vi "日志信息出发送队列 (子VI).vi"(11 "queue out":refnum<queue>) -> (0 "错误输出":errorcluster)   [LabVIEW 2016, in "数据传输系统-03.lvlib"]
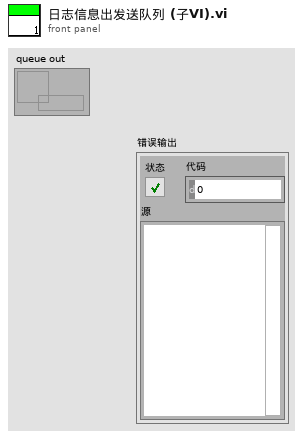
[diagram p1: front panel]
types:
  T1 = enum16{"空白测试", "跨度核查", "标样核查", "加标回收", "平行样", "集成干预"}
  T2 = typedef "数据传输系统-03.lvlib/应用环境.ctl" = enum16{"STD", "GB212", "婉仪平台"}
  T3 = cluster{"氨氮零点核查索引起始时间":string, "总磷零点核查索引起始时间":string, "总氮零点核查索引起始时间":string, "CODMn零点核查索引起始时间":string, "CODCr零点核查索引起始时间":string, "亚硝酸盐零点核查索引起始时间":string, "硫化物零点核查索引起始时间":string, "ORP零点核查索引起始时间":string, "氟化物零点核查索引起始时间":string, "挥发酚零点核查索引起始时间":string}
  T4 = cluster{"数组[0]":string, "数组[1]":string, "数组[2]":string, "数组[3]":string, "数组[4]":string, "数组[5]":string, "数组[6]":string, "数组[7]":string, "数组[8]":string, "数组[9]":string}
  T5 = cluster{"PH":string[][], "CODCr":string[][], "氨氮":string[][], "CODMn":string[][], "总氮":string[][], "总磷":string[][], "电导率":string[][], "水温":string[][], "COD":string[][], "DO":string[][], "浊度":string[][], "叶绿素":string[][], "藻密度":string[][], "铜":string[][], "盐度":string[][], "水位":string[][], "流速":string[][], "方向":string[][], "瞬时流量":string[][], "累积流量":string[][], "正累积流量":string[][], "负累积流量":string[][], "亚硝酸盐":string[][], "硫化物":string[][], "ORP":string[][], "铅":string[][], "镉":string[][], "锌":string[][], "镍":string[][], "锰":string[][], "汞":string[][], "气温":string[][], "气压":string[][], "风速":string[][], "风向":string[][], "空气温度":string[][], "相对湿度":string[][], "分钟雨量":string[][], "小时雨量":string[][], "日雨量":string[][], "累积雨量":string[][], "盐度":string[][], "磷酸盐":string[][], "硝氮":string[][], "氟化物":string[][], "挥发酚":string[][], "氯化物":string[][], "蓝绿藻":string[][], "余氯":string[][], "综合生物毒性":string[][], "水深":string[][]}
  T6 = cluster{"氨氮跨度核查索引起始时间":string, "总磷跨度核查索引起始时间":string, "总氮跨度核查索引起始时间":string, "CODMn跨度核查索引起始时间":string, "CODCr跨度核查索引起始时间":string, "亚硝酸盐跨度核查索引起始时间":string, "硫化物跨度核查索引起始时间":string, "ORP跨度核查索引起始时间":string, "氟化物跨度核查索引起始时间":string, "挥发酚跨度核查索引起始时间":string}
  T7 = cluster{"氨氮标样核查索引起始时间":string, "总磷标样核查索引起始时间":string, "总氮标样核查索引起始时间":string, "CODMn标样核查索引起始时间":string, "CODCr标样核查索引起始时间":string, "DO标样核查索引起始时间":string, "PH标样核查索引起始时间":string, "比电导率标样核查索引起始时间":string, "水温标样核查索引起始时间":string, "浊度标样核查索引起始时间":string, "叶绿素a标样核查索引起始时间":string, "藻密度标样核查索引起始时间":string, "亚硝酸盐标样核查索引起始时间":string, "硫化物标样核查索引起始时间":string, "ORP标样核查索引起始时间":string, "氟化物标样核查索引起始时间":string, "挥发酚标样核查索引起始时间":string, "氯化物标样核查索引起始时间":string}
  T8 = cluster{"数组[0]":string, "数组[1]":string, "数组[2]":string, "数组[3]":string, "数组[4]":string, "数组[5]":string, "数组[6]":string, "数组[7]":string, "数组[8]":string, "数组[9]":string, "数组[10]":string, "数组[11]":string, "数组[12]":string, "数组[13]":string, "数组[14]":string, "数组[15]":string, "数组[16]":string, "数组[17]":string}
  T9 = cluster{"氨氮加标回收索引起始时间":string, "总磷加标回收索引起始时间":string, "总氮加标回收索引起始时间":string, "CODMn加标回收索引起始时间":string, "CODCr加标回收索引起始时间":string, "氟化物加标回收索引起始时间":string, "挥发酚加标回收索引起始时间":string}
  T10 = cluster{"[0]":string, "[1]":string, "[2]":string, "[3]":string, "[4]":string, "[5]":string, "[6]":string}
  T11 = cluster{"氨氮平行样索引起始时间":string, "总磷平行样索引起始时间":string, "总氮平行样索引起始时间":string, "CODMn平行样索引起始时间":string, "CODCr平行样索引起始时间":string, "氟化物平行样索引起始时间":string, "挥发酚平行样索引起始时间":string}
  T12 = cluster{"氨氮集成干预索引起始时间":string, "总磷集成干预索引起始时间":string, "总氮集成干预索引起始时间":string, "CODMn集成干预索引起始时间":string, "CODCr集成干预索引起始时间":string, "DO集成干预索引起始时间":string, "PH集成干预索引起始时间":string, "比电导率集成干预索引起始时间":string, "水温集成干预索引起始时间":string, "浊度集成干预索引起始时间":string, "叶绿素a集成干预索引起始时间":string, "藻密度集成干预索引起始时间":string, "亚硝酸盐集成干预索引起始时间":string, "硫化物集成干预索引起始时间":string, "ORP集成干预索引起始时间":string, "氟化物集成干预索引起始时间":string, "挥发酚集成干预索引起始时间":string, "氯化物集成干预索引起始时间":string}
  T13 = cluster{"[0]":string, "[1]":string, "[2]":string, "[3]":string, "[4]":string, "[5]":string, "[6]":string, "[7]":string, "[8]":string, "[9]":string, "[10]":string, "[11]":string, "[12]":string, "[13]":string, "[14]":string, "[15]":string, "[16]":string, "[17]":string}
  T14 = cluster{"氨氮仪器日志索引起始时间":string, "总磷仪器日志索引起始时间":string, "总氮仪器日志索引起始时间":string, "CODMn仪器日志索引起始时间":string, "CODCr仪器日志索引起始时间":string, "系统仪器日志索引起始时间":string, "氟化物仪器日志索引起始时间":string, "挥发酚仪器日志索引起始时间":string}
  T15 = cluster{"[0]":string, "[1]":string, "[2]":string, "[3]":string, "[4]":string, "[5]":string, "[6]":string, "[7]":string}
  T16 = cluster{"氨氮报警信息索引起始时间":string, "总磷报警信息索引起始时间":string, "总氮报警信息索引起始时间":string, "CODMn报警信息索引起始时间":string, "CODCr报警信息索引起始时间":string, "DO报警信息索引起始时间":string, "PH报警信息索引起始时间":string, "比电导率报警信息索引起始时间":string, "水温报警信息索引起始时间":string, "浊度报警信息索引起始时间":string, "叶绿素报警信息索引起始时间":string, "系统报警信息索引起始时间":string, "氟化物报警信息索引起始时间":string, "挥发酚报警信息索引起始时间":string}
  T17 = cluster{"[0]":string, "[1]":string, "[2]":string, "[3]":string, "[4]":string, "[5]":string, "[6]":string, "[7]":string, "[8]":string, "[9]":string, "[10]":string, "[11]":string, "[12]":string, "[13]":string}
  T18 = cluster{"氨氮仪器参数索引起始时间":string, "总磷仪器参数索引起始时间":string, "总氮仪器参数索引起始时间":string, "CODMn仪器参数索引起始时间":string, "CODCr仪器参数索引起始时间":string, "DO仪器参数索引起始时间":string, "PH仪器参数索引起始时间":string, "比电导率仪器参数索引起始时间":string, "水温仪器参数索引起始时间":string, "浊度仪器参数索引起始时间":string, "叶绿素a仪器参数索引起始时间":string, "藻密度仪器参数索引起始时间":string, "ORP仪器参数索引起始时间":string, "氟化物仪器参数索引起始时间":string, "挥发酚仪器参数索引起始时间":string}
  T19 = cluster{"[0]":string, "[1]":string, "[2]":string, "[3]":string, "[4]":string, "[5]":string, "[6]":string, "[7]":string, "[8]":string, "[9]":string, "[10]":string, "[11]":string, "[12]":string, "[13]":string, "[14]":string}
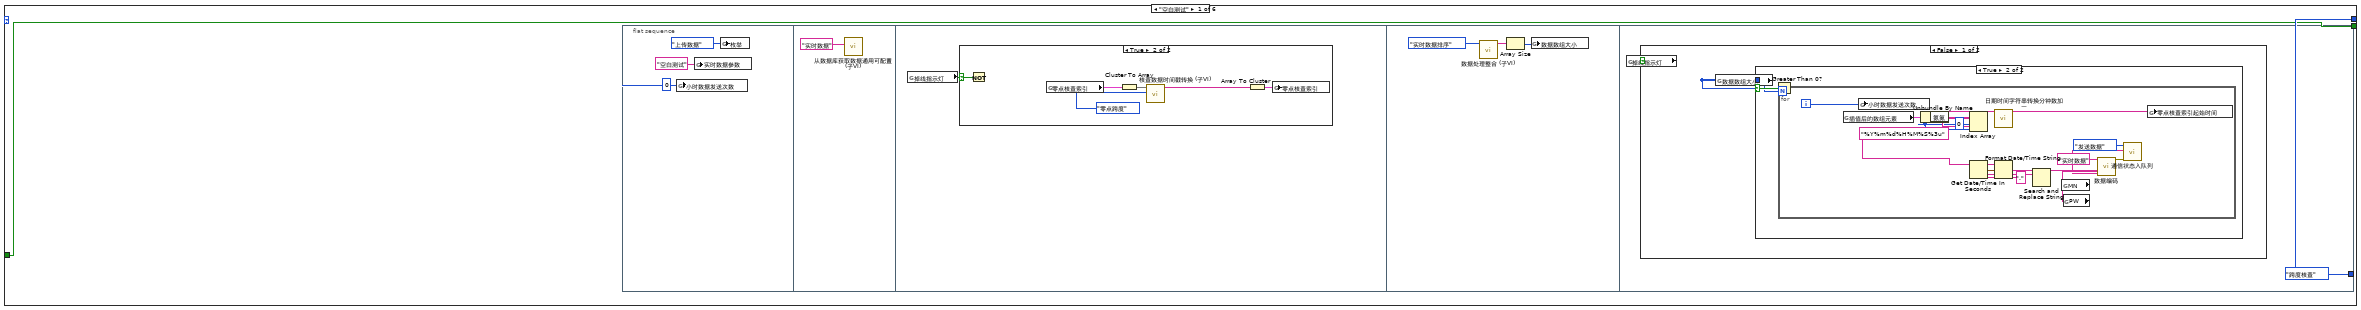
[diagram p2: hidden frame]
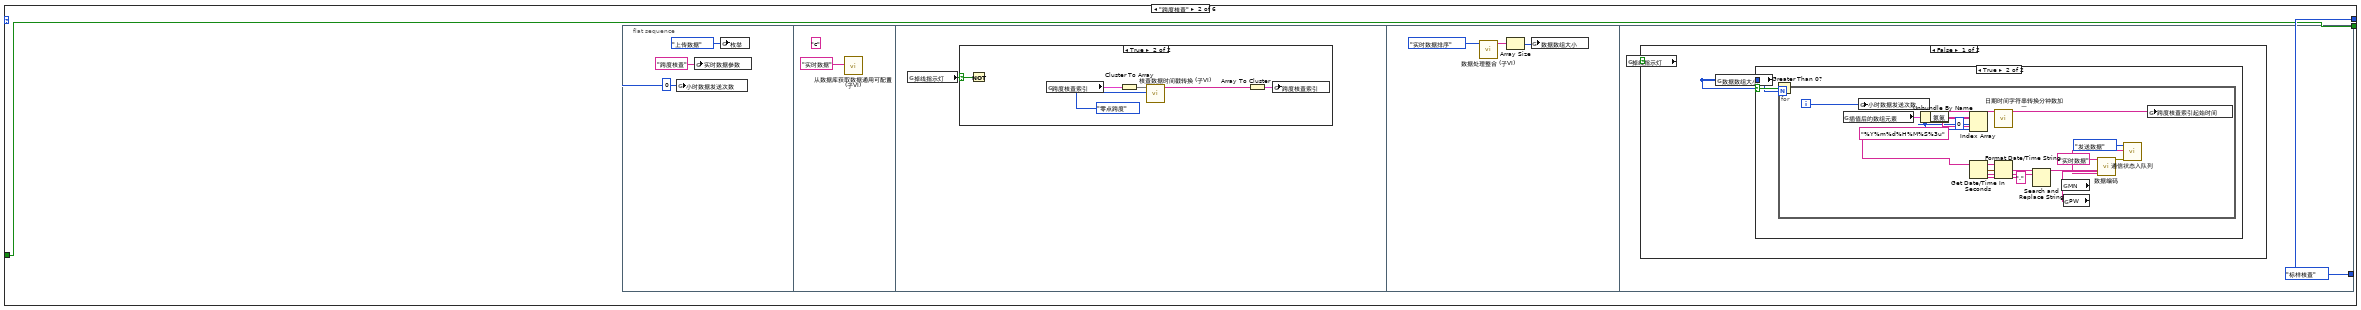
[diagram p6: hidden frame]
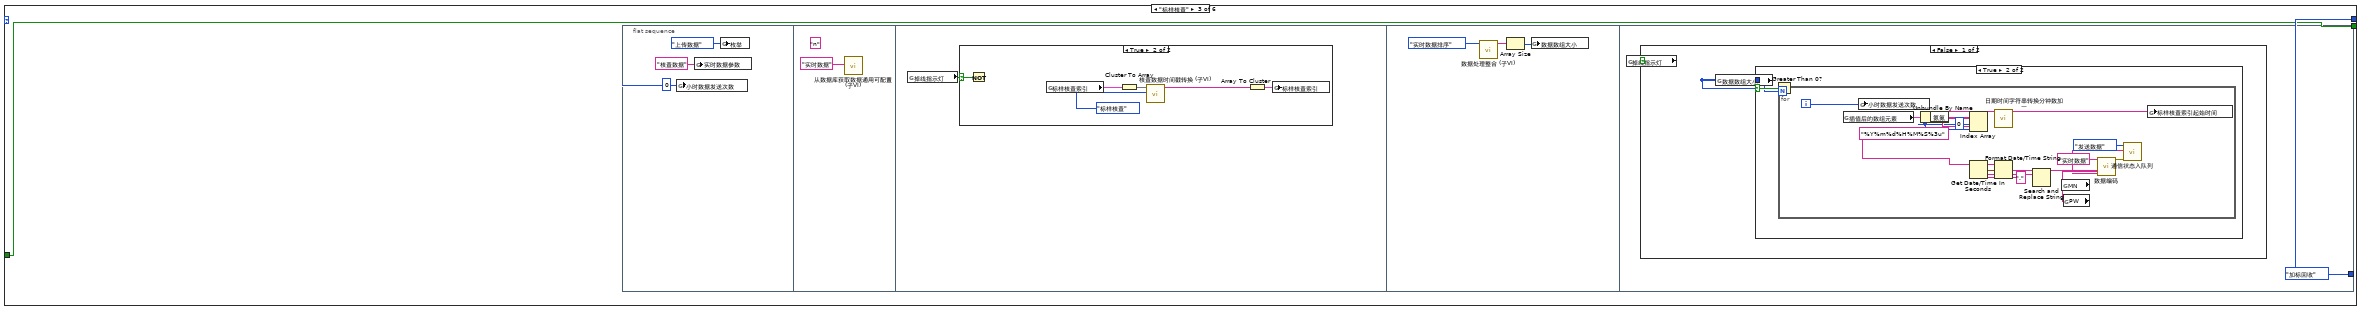
[diagram p10: hidden frame]
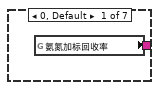
[diagram p15: hidden frame]
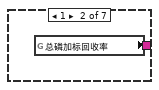
[diagram p16: hidden frame]
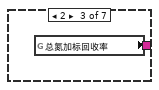
[diagram p17: hidden frame]
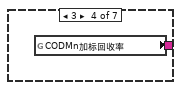
[diagram p18: hidden frame]
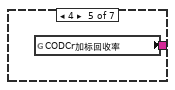
[diagram p19: hidden frame]
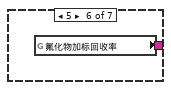
[diagram p20: hidden frame]
diagram:
  n1 = while "While循环" {
    shift-right: [w12] -> _
    shift-left: "质控数据" ("组合框") -> [w13]
    tunnel: [errorcluster {"status"=FALSE, "code"=0, "source"=""} ("错误输出")] -> w3
    tunnel: "queue out" -> [w9]
    stop <- w10 stop-if-true
    # "所有的主动上传数据都是有数据才会上传"
    n2 = Get Queue Status(queue=w9, return elements? (F)=TRUE ("返回元素？(F)")) -> (elements=w8:string[])  [unwired: 1 in, 7 out]
    n3 = Index Array(array=w8) -> (element=w7:string)  [unwired: 1 in]
    n4 = Equal?(x=w7, y="反控命令" ("元素")) -> (x = y?=w5:bool)
    n5 = case shown="\"质控数据\"" w13 {
      tunnel: [w23 w328 "系统状态" ("组合框") w431 "测量周期" ("组合框") "超标留样" ("组合框") "报警信息" ("组合框") w576 w643 "环境参数" ("组合框") "环境参数" ("组合框")] -> w12
      tunnel: [w14 w327 w385 w429 w455 w489 w554 w575 w642 w689 TRUE] -> w10
      tunnel: w5 -> [w14 w327 w385 w429 w455 w489 w554 w575 w642 w689 _]
      frame "质控数据" {
        n6 = global read "断电保存全局.vi" "数据组合发送"() -> (w18:bool)
        n7 = global read "断电保存全局.vi" "数据发送协议"() -> (w21:enum16{"2005-212协议", "2017-212协议"})
        n8 = Not(x=w18) -> (.not. x?=w17:bool)
        n9 = Equal?(x=w21, y=enum16{"2005-212协议", "2017-212协议"}."2017-212协议" ("数据发送协议")) -> (x = y?=w19:bool)
        n10 = And(x=w17, y=w19) -> (x .and. y?=w16:bool)
        n11 = case shown="True" w16 {
          tunnel: [T1."空白测试" T1."加标回收"] -> w15
          frame False {
          }
          frame True {
          }
        }
        n12 = while {
          shift-right: [w27] -> _
          shift-left: w15 -> [w28]
          tunnel: w14 -> [w24]
          stop <- w25 stop-if-true
          n13 = case shown="\"加标回收\"" w28 {
            tunnel: [w29 w67 w105 w143 w204 TRUE] -> w25
            tunnel: [w30 w68 w106 w144 w205 w258] -> w27
            tunnel: w24 -> [w29 w67 w105 w143 w204 _]
            frame "空白测试" {
              n14 = flat-sequence {
                tunnel: [T1."跨度核查"] -> w30
                frame #0 {
                  n15 = global write "全局 小时数据发送次数.vi" "小时数据发送次数"(0 ("小时数据发送次数")) -> ()
                  n16 = global write "全局 实时数据参数.vi" "实时数据参数"("空白测试") -> ()
                  n17 = global write "全局1.vi" "枚举"(enum16{"返回请求应答", "上传数据", "返回执行结果"}."上传数据" ("枚举")) -> ()
                }
                frame #1 {
                  n18 = call "从数据库获取数据通用可配置(子VI).vi"("table输入"="实时数据" ("新元素/子数组")) -> ()  [unwired: 9 in, 2 out]
                }
                frame #2 {
                  n19 = global read "全局 数据发送重叠.vi" "掉线指示灯"() -> (w36:bool)
                  n20 = Not(x=w36) -> (.not. x?=w35:bool)
                  n21 = case shown="True" w35 {
                    frame False {
                    }
                    frame True {
                      n22 = global read "全局 时间2.vi" "零点核查索引"() -> (w41:T3)
                      n23 = Cluster To Array(cluster=w41) -> (array=w39:string[])
                      n24 = call "核查数据时间戳转换 (子VI).vi"("枚举"=enum16{"零点跨度", "标样核查"}."零点跨度", "核查索引"=w39) -> ("数组"=w38:string[])  [unwired: 9 in]
                      n25 = Array To Cluster(array=w38) -> (cluster=w40:T4)
                      n26 = global write "全局 时间2.vi" "零点核查索引"(w40) -> ()
                    }
                  }
                }
                frame #3 {
                  n27 = call "数据处理整合 (子VI).vi"("枚举"=enum16{"实时数据排序", "小时数据排序"}."实时数据排序") -> ("已排序的数组"=w44:string[])  [unwired: 10 in]
                  n28 = Array Size(array=w44) -> (size(s)=w43:i32)
                  n29 = global write "全局 数据数组大小.vi" "数据数组大小"(w43) -> ()
                }
                frame #4 {
                  n30 = global read "全局 数据发送重叠.vi" "掉线指示灯"() -> (w46:bool)
                  n31 = case shown="False" w46 {
                    frame False {
                      n32 = global read "全局 数据数组大小.vi" "数据数组大小"() -> (w47:i32)
                      n33 = Greater Than 0?(x=w47) -> (x > 0?=w48:bool)
                      n34 = case shown="True" w48 {
                        tunnel: w47 -> [_ w49]
                        frame False {
                        }
                        frame True {
                          n35 = for {
                            N: w49 -> [_]
                            i -> [w52]
                            w61 = 0 ("禁用的索引 (列)")
                            n36 = global read "插值后的新数组.vi" "插值后的数组元素"() -> (w65:T5)
                            n37 = global write "全局 小时数据发送次数.vi" "小时数据发送次数"(w52) -> ()
                            n38 = Unbundle By Name(w65) -> ("氨氮"=w64:string[][])
                            n39 = Index Array(array=w64, index (row)=w61, index (col)=w61) -> (element=w63:string)
                            n40 = Get Date/Time In Seconds() -> (seconds since 1Jan1904=w56:timestamp)
                            n41 = call "日期时间字符串转换分钟数加一.vi"("data[0]"=w63) -> ("日期/时间字符串"=w62:string)  [unwired: 10 in]
                            n42 = Format Date/Time String(time format string (%c)="%Y%m%d%H%M%S%3u" ("时间格式字符串(%c)"), seconds (now)=w56) -> (date/time string=w55:string)  [unwired: 1 in]
                            n43 = Search and Replace String(input string=w55, search string="." ("搜索字符串")) -> (result string=w53:string)  [unwired: 6 in, 3 out]
                            n44 = global read "断电保存全局.vi" "MN"() -> (w60:string)
                            n45 = global read "断电保存全局.vi" "PW"() -> (w59:string)
                            n46 = call "数据编码.vi"("table输入"="实时数据" ("新元素/子数组"), "QN"=w53, "MN"=w60, "PW"=w59) -> ("错误常量"=w58:errorcluster, "通讯包字符串"=w50:string)  [unwired: 10 in]
                            n47 = call "通信状态入队列.vi"("错误输入（无错误）"=w58, "发送报文"=w50, "枚举"=enum16{"打开连接", "发送数据", "读取数据", "数据处理", "关闭连接"}."发送数据") -> ()  [unwired: 8 in, 1 out]
                            n48 = global write "全局 时间2.vi" "零点核查索引起始时间"(w62) -> ()
                          }
                        }
                      }
                    }
                    frame True {
                    }
                  }
                }
              }
            }
            frame "跨度核查" {
              n49 = flat-sequence {
                tunnel: [T1."标样核查"] -> w68
                frame #0 {
                  n50 = global write "全局 小时数据发送次数.vi" "小时数据发送次数"(0 ("小时数据发送次数")) -> ()
                  n51 = global write "全局 实时数据参数.vi" "实时数据参数"("跨度核查") -> ()
                  n52 = global write "全局1.vi" "枚举"(enum16{"返回请求应答", "上传数据", "返回执行结果"}."上传数据" ("枚举")) -> ()
                }
                frame #1 {
                  (unwired) "c" ("列队名（唯一）")
                  n53 = call "从数据库获取数据通用可配置(子VI).vi"("table输入"="实时数据" ("新元素/子数组")) -> ()  [unwired: 9 in, 2 out]
                }
                frame #2 {
                  n54 = global read "全局 数据发送重叠.vi" "掉线指示灯"() -> (w74:bool)
                  n55 = Not(x=w74) -> (.not. x?=w73:bool)
                  n56 = case shown="True" w73 {
                    frame False {
                    }
                    frame True {
                      n57 = global read "全局 时间2.vi" "跨度核查索引"() -> (w79:T6)
                      n58 = Cluster To Array(cluster=w79) -> (array=w77:string[])
                      n59 = call "核查数据时间戳转换 (子VI).vi"("枚举"=enum16{"零点跨度", "标样核查"}."零点跨度", "核查索引"=w77) -> ("数组"=w76:string[])  [unwired: 9 in]
                      n60 = Array To Cluster(array=w76) -> (cluster=w78:T4)
                      n61 = global write "全局 时间2.vi" "跨度核查索引"(w78) -> ()
                    }
                  }
                }
                frame #3 {
                  n62 = call "数据处理整合 (子VI).vi"("枚举"=enum16{"实时数据排序", "小时数据排序"}."实时数据排序") -> ("已排序的数组"=w82:string[])  [unwired: 10 in]
                  n63 = Array Size(array=w82) -> (size(s)=w81:i32)
                  n64 = global write "全局 数据数组大小.vi" "数据数组大小"(w81) -> ()
                }
                frame #4 {
                  n65 = global read "全局 数据发送重叠.vi" "掉线指示灯"() -> (w84:bool)
                  n66 = case shown="False" w84 {
                    frame False {
                      n67 = global read "全局 数据数组大小.vi" "数据数组大小"() -> (w85:i32)
                      n68 = Greater Than 0?(x=w85) -> (x > 0?=w86:bool)
                      n69 = case shown="True" w86 {
                        tunnel: w85 -> [_ w87]
                        frame False {
                        }
                        frame True {
                          n70 = for {
                            N: w87 -> [_]
                            i -> [w90]
                            w99 = 0 ("禁用的索引 (列)")
                            n71 = global read "插值后的新数组.vi" "插值后的数组元素"() -> (w103:T5)
                            n72 = global write "全局 小时数据发送次数.vi" "小时数据发送次数"(w90) -> ()
                            n73 = Unbundle By Name(w103) -> ("氨氮"=w102:string[][])
                            n74 = Index Array(array=w102, index (row)=w99, index (col)=w99) -> (element=w101:string)
                            n75 = Get Date/Time In Seconds() -> (seconds since 1Jan1904=w94:timestamp)
                            n76 = call "日期时间字符串转换分钟数加一.vi"("data[0]"=w101) -> ("日期/时间字符串"=w100:string)  [unwired: 10 in]
                            n77 = Format Date/Time String(time format string (%c)="%Y%m%d%H%M%S%3u" ("时间格式字符串(%c)"), seconds (now)=w94) -> (date/time string=w93:string)  [unwired: 1 in]
                            n78 = Search and Replace String(input string=w93, search string="." ("搜索字符串")) -> (result string=w91:string)  [unwired: 6 in, 3 out]
                            n79 = global read "断电保存全局.vi" "MN"() -> (w98:string)
                            n80 = global read "断电保存全局.vi" "PW"() -> (w97:string)
                            n81 = call "数据编码.vi"("table输入"="实时数据" ("新元素/子数组"), "QN"=w91, "MN"=w98, "PW"=w97) -> ("错误常量"=w96:errorcluster, "通讯包字符串"=w88:string)  [unwired: 10 in]
                            n82 = call "通信状态入队列.vi"("错误输入（无错误）"=w96, "发送报文"=w88, "枚举"=enum16{"打开连接", "发送数据", "读取数据", "数据处理", "关闭连接"}."发送数据") -> ()  [unwired: 8 in, 1 out]
                            n83 = global write "全局 时间2.vi" "跨度核查索引起始时间"(w100) -> ()
                          }
                        }
                      }
                    }
                    frame True {
                    }
                  }
                }
              }
            }
            frame "标样核查" {
              n84 = flat-sequence {
                tunnel: [T1."加标回收"] -> w106
                frame #0 {
                  n85 = global write "全局 小时数据发送次数.vi" "小时数据发送次数"(0 ("小时数据发送次数")) -> ()
                  n86 = global write "全局 实时数据参数.vi" "实时数据参数"("核查数据") -> ()
                  n87 = global write "全局1.vi" "枚举"(enum16{"返回请求应答", "上传数据", "返回执行结果"}."上传数据" ("枚举")) -> ()
                }
                frame #1 {
                  (unwired) "n" ("列队名（唯一）")
                  n88 = call "从数据库获取数据通用可配置(子VI).vi"("table输入"="实时数据" ("新元素/子数组")) -> ()  [unwired: 9 in, 2 out]
                }
                frame #2 {
                  n89 = global read "全局 数据发送重叠.vi" "掉线指示灯"() -> (w112:bool)
                  n90 = Not(x=w112) -> (.not. x?=w111:bool)
                  n91 = case shown="True" w111 {
                    frame False {
                    }
                    frame True {
                      n92 = global read "全局 时间2.vi" "标样核查索引"() -> (w117:T7)
                      n93 = Cluster To Array(cluster=w117) -> (array=w115:string[])
                      n94 = call "核查数据时间戳转换 (子VI).vi"("枚举"=enum16{"零点跨度", "标样核查"}."标样核查", "核查索引"=w115) -> ("数组"=w114:string[])  [unwired: 9 in]
                      n95 = Array To Cluster(array=w114) -> (cluster=w116:T8)
                      n96 = global write "全局 时间2.vi" "标样核查索引"(w116) -> ()
                    }
                  }
                }
                frame #3 {
                  n97 = call "数据处理整合 (子VI).vi"("枚举"=enum16{"实时数据排序", "小时数据排序"}."实时数据排序") -> ("已排序的数组"=w120:string[])  [unwired: 10 in]
                  n98 = Array Size(array=w120) -> (size(s)=w119:i32)
                  n99 = global write "全局 数据数组大小.vi" "数据数组大小"(w119) -> ()
                }
                frame #4 {
                  n100 = global read "全局 数据发送重叠.vi" "掉线指示灯"() -> (w122:bool)
                  n101 = case shown="False" w122 {
                    frame False {
                      n102 = global read "全局 数据数组大小.vi" "数据数组大小"() -> (w123:i32)
                      n103 = Greater Than 0?(x=w123) -> (x > 0?=w124:bool)
                      n104 = case shown="True" w124 {
                        tunnel: w123 -> [_ w125]
                        frame False {
                        }
                        frame True {
                          n105 = for {
                            N: w125 -> [_]
                            i -> [w128]
                            w137 = 0 ("禁用的索引 (列)")
                            n106 = global read "插值后的新数组.vi" "插值后的数组元素"() -> (w141:T5)
                            n107 = global write "全局 小时数据发送次数.vi" "小时数据发送次数"(w128) -> ()
                            n108 = Unbundle By Name(w141) -> ("氨氮"=w140:string[][])
                            n109 = Index Array(array=w140, index (row)=w137, index (col)=w137) -> (element=w139:string)
                            n110 = Get Date/Time In Seconds() -> (seconds since 1Jan1904=w132:timestamp)
                            n111 = call "日期时间字符串转换分钟数加一.vi"("data[0]"=w139) -> ("日期/时间字符串"=w138:string)  [unwired: 10 in]
                            n112 = Format Date/Time String(time format string (%c)="%Y%m%d%H%M%S%3u" ("时间格式字符串(%c)"), seconds (now)=w132) -> (date/time string=w131:string)  [unwired: 1 in]
                            n113 = Search and Replace String(input string=w131, search string="." ("搜索字符串")) -> (result string=w129:string)  [unwired: 6 in, 3 out]
                            n114 = global read "断电保存全局.vi" "MN"() -> (w136:string)
                            n115 = global read "断电保存全局.vi" "PW"() -> (w135:string)
                            n116 = call "数据编码.vi"("table输入"="实时数据" ("新元素/子数组"), "QN"=w129, "MN"=w136, "PW"=w135) -> ("错误常量"=w134:errorcluster, "通讯包字符串"=w126:string)  [unwired: 10 in]
                            n117 = call "通信状态入队列.vi"("错误输入（无错误）"=w134, "发送报文"=w126, "枚举"=enum16{"打开连接", "发送数据", "读取数据", "数据处理", "关闭连接"}."发送数据") -> ()  [unwired: 8 in, 1 out]
                            n118 = global write "全局 时间2.vi" "标样核查索引起始时间"(w138) -> ()
                          }
                        }
                      }
                    }
                    frame True {
                    }
                  }
                }
              }
            }
            frame "加标回收" {
              n119 = flat-sequence {
                tunnel: [T1."平行样"] -> w144
                frame #0 {
                  n120 = global write "全局 小时数据发送次数.vi" "小时数据发送次数"(0 ("小时数据发送次数")) -> ()
                  n121 = global write "全局1.vi" "枚举"(enum16{"返回请求应答", "上传数据", "返回执行结果"}."上传数据" ("枚举")) -> ()
                  n122 = global write "全局 实时数据参数.vi" "实时数据参数"("加标回收测试") -> ()
                }
                frame #1 {
                  (unwired) "d" ("列队名（唯一）")
                  n123 = call "从数据库获取数据通用可配置(子VI).vi"("table输入"="加标回收" ("新元素/子数组")) -> ()  [unwired: 9 in, 2 out]
                }
                frame #2 {
                  n124 = global read "全局 数据发送重叠.vi" "掉线指示灯"() -> (w150:bool)
                  n125 = Not(x=w150) -> (.not. x?=w149:bool)
                  n126 = case shown="True" w149 {
                    frame False {
                    }
                    frame True {
                      n127 = global read "全局 时间2.vi" "加标回收索引"() -> (w154:T9)
                      n128 = Cluster To Array(cluster=w154) -> (array=w153:string[])
                      n129 = for {
                        tunnel: [w156] -> w151 mode=indexing
                        tunnel: w153 -> [w155] mode=indexing
                        i -> [w157]
                        # "行数大于零"
                        n130 = case shown="6" w157 {
                          tunnel: [w162 w163 w164 w165 w166 w167 w168] -> w158
                          frame 0, Default {
                            n131 = global read "全局 所有参数.vi" "氨氮加标回收率"() -> (w162:string[][])
                          }
                          frame 1 {
                            n132 = global read "全局 所有参数.vi" "总磷加标回收率"() -> (w163:string[][])
                          }
                          frame 2 {
                            n133 = global read "全局 所有参数.vi" "总氮加标回收率"() -> (w164:string[][])
                          }
                          frame 3 {
                            n134 = global read "全局 所有参数.vi" "CODMn加标回收率"() -> (w165:string[][])
                          }
                          frame 4 {
                            n135 = global read "全局 所有参数.vi" "CODCr加标回收率"() -> (w166:string[][])
                          }
                          frame 5 {
                            n136 = global read "全局 所有参数.vi" "氟化物加标回收率"() -> (w167:string[][])
                          }
                          frame 6 {
                            n137 = global read "全局 所有参数.vi" "挥发酚加标回收率"() -> (w168:string[][])
                          }
                        }
                        n138 = Array Size(array=w158) -> (size(s)=w160:i32[])
                        n139 = Index Array(array=w160) -> (element=w159:i32)  [unwired: 1 in]
                        n140 = Greater Than 0?(x=w159) -> (x > 0?=w161:bool)
                        n141 = case shown="True" w161 {
                          tunnel: w157 -> [_ _]
                          tunnel: w159 -> [_ _]
                          tunnel: w158 -> [_ w173]
                          tunnel: [w169 w170] -> w156
                          tunnel: w155 -> [w169 _]
                          frame False {
                          }
                          frame True {
                            # "最新时间戳加1分钟"
                            n142 = Array Size(array=w173) -> (size(s)=w175:i32[])
                            n143 = Index Array(array=w175) -> (element=w174:i32)  [unwired: 1 in]
                            n144 = Decrement(x=w174) -> (x-1=w172:i32)
                            n145 = Index Array(array=w173, index (row)=w172, index (col)=0 ("禁用的索引 (列)")) -> (element=w176:string)
                            n146 = call "日期时间字符串转换分钟数加一.vi"("data[0]"=w176) -> ("日期/时间字符串"=w170:string)  [unwired: 10 in]
                          }
                        }
                      }
                      n147 = Array To Cluster(array=w151) -> (cluster=w152:T10)
                      n148 = global write "全局 时间2.vi" "加标回收索引"(w152) -> ()
                    }
                  }
                }
                frame #3 {
                  n149 = call "加标回收数据处理整合 (子VI).vi"("枚举"=enum16{"实时数据排序", "小时数据排序"}."实时数据排序") -> ("已排序的数组"=w178:string[])  [unwired: 10 in]
                  n150 = Array Size(array=w178) -> (size(s)=w179:i32)
                  n151 = global write "全局 数据数组大小.vi" "数据数组大小"(w179) -> ()
                }
                frame #4 {
                  n152 = global read "全局 数据发送重叠.vi" "掉线指示灯"() -> (w181:bool)
                  n153 = case shown="False" w181 {
                    frame False {
                      n154 = global read "全局 数据数组大小.vi" "数据数组大小"() -> (w182:i32)
                      n155 = Greater Than 0?(x=w182) -> (x > 0?=w183:bool)
                      n156 = case shown="True" w183 {
                        tunnel: w182 -> [_ w184]
                        frame False {
                        }
                        frame True {
                          n157 = for {
                            N: w184 -> [_]
                            i -> [w187]
                            n158 = global read "插值后的新数组.vi" "插值后的数组元素"() -> (w202:T5)
                            n159 = global read "全局 数据数组大小.vi" "数据数组大小"() -> (w199:i32)
                            n160 = global write "全局 小时数据发送次数.vi" "小时数据发送次数"(w187) -> ()
                            n161 = Unbundle By Name(w202) -> ("氨氮"=w201:string[][])
                            n162 = Decrement(x=w199) -> (x-1=w198:i32)
                            n163 = Index Array(array=w201, index (row)=w198, index (col)=0 ("禁用的索引 (列)")) -> (element=w197:string)
                            n164 = Get Date/Time In Seconds() -> (seconds since 1Jan1904=w191:timestamp)
                            n165 = call "日期时间字符串转换分钟数加一.vi"("data[0]"=w197) -> ("日期/时间字符串"=w196:string)  [unwired: 10 in]
                            n166 = Format Date/Time String(time format string (%c)="%Y%m%d%H%M%S%3u" ("时间格式字符串(%c)"), seconds (now)=w191) -> (date/time string=w190:string)  [unwired: 1 in]
                            n167 = Search and Replace String(input string=w190, search string="." ("搜索字符串")) -> (result string=w188:string)  [unwired: 6 in, 3 out]
                            n168 = global read "断电保存全局.vi" "MN"() -> (w195:string)
                            n169 = global read "断电保存全局.vi" "PW"() -> (w194:string)
                            n170 = call "数据编码.vi"("table输入"="实时数据" ("新元素/子数组"), "QN"=w188, "MN"=w195, "PW"=w194) -> ("错误常量"=w193:errorcluster, "通讯包字符串"=w185:string)  [unwired: 10 in]
                            n171 = call "通信状态入队列.vi"("错误输入（无错误）"=w193, "发送报文"=w185, "枚举"=enum16{"打开连接", "发送数据", "读取数据", "数据处理", "关闭连接"}."发送数据") -> ()  [unwired: 8 in, 1 out]
                            n172 = global write "全局 时间2.vi" "加标回收索引起始时间"(w196) -> ()
                          }
                        }
                      }
                    }
                    frame True {
                    }
                  }
                }
              }
            }
            frame "平行样" {
              n173 = flat-sequence {
                tunnel: [T1."集成干预"] -> w205
                frame #0 {
                  n174 = global write "全局 小时数据发送次数.vi" "小时数据发送次数"(0 ("小时数据发送次数")) -> ()
                  n175 = global write "全局1.vi" "枚举"(enum16{"返回请求应答", "上传数据", "返回执行结果"}."上传数据" ("枚举")) -> ()
                  n176 = global write "全局 实时数据参数.vi" "实时数据参数"("平行样测试") -> ()
                }
                frame #1 {
                  (unwired) "e" ("列队名（唯一）")
                  n177 = call "从数据库获取数据通用可配置(子VI).vi"("table输入"="平行样测试" ("新元素/子数组")) -> ()  [unwired: 9 in, 2 out]
                }
                frame #2 {
                  n178 = global read "全局 数据发送重叠.vi" "掉线指示灯"() -> (w211:bool)
                  n179 = Not(x=w211) -> (.not. x?=w210:bool)
                  n180 = case shown="True" w210 {
                    frame False {
                    }
                    frame True {
                      n181 = global read "全局 时间2.vi" "平行样索引"() -> (w215:T11)
                      n182 = Cluster To Array(cluster=w215) -> (array=w214:string[])
                      n183 = for {
                        tunnel: [w217] -> w212 mode=indexing
                        tunnel: w214 -> [w216] mode=indexing
                        i -> [w218]
                        # "行数大于零"
                        n184 = case shown="6" w218 {
                          tunnel: [w223 w224 w225 w226 w227 w228 w229] -> w219
                          frame 0, Default {
                            n185 = global read "全局 所有参数.vi" "氨氮"() -> (w223:string[][])
                          }
                          frame 1 {
                            n186 = global read "全局 所有参数.vi" "总磷"() -> (w224:string[][])
                          }
                          frame 2 {
                            n187 = global read "全局 所有参数.vi" "总氮"() -> (w225:string[][])
                          }
                          frame 3 {
                            n188 = global read "全局 所有参数.vi" "CODMn"() -> (w226:string[][])
                          }
                          frame 4 {
                            n189 = global read "全局 所有参数.vi" "CODCr"() -> (w227:string[][])
                          }
                          frame 5 {
                            n190 = global read "全局 所有参数.vi" "氟化物"() -> (w228:string[][])
                          }
                          frame 6 {
                            n191 = global read "全局 所有参数.vi" "挥发酚"() -> (w229:string[][])
                          }
                        }
                        n192 = Array Size(array=w219) -> (size(s)=w221:i32[])
                        n193 = Index Array(array=w221) -> (element=w220:i32)  [unwired: 1 in]
                        n194 = Greater Than 0?(x=w220) -> (x > 0?=w222:bool)
                        n195 = case shown="True" w222 {
                          tunnel: w218 -> [_ _]
                          tunnel: w220 -> [_ _]
                          tunnel: w219 -> [_ w234]
                          tunnel: [w230 w231] -> w217
                          tunnel: w216 -> [w230 _]
                          frame False {
                          }
                          frame True {
                            # "最新时间戳加1分钟"
                            n196 = Array Size(array=w234) -> (size(s)=w236:i32[])
                            n197 = Index Array(array=w236) -> (element=w235:i32)  [unwired: 1 in]
                            n198 = Decrement(x=w235) -> (x-1=w233:i32)
                            n199 = Index Array(array=w234, index (row)=w233, index (col)=0 ("禁用的索引 (列)")) -> (element=w237:string)
                            n200 = call "日期时间字符串转换分钟数加一.vi"("data[0]"=w237) -> ("日期/时间字符串"=w231:string)  [unwired: 10 in]
                          }
                        }
                      }
                      n201 = Array To Cluster(array=w212) -> (cluster=w213:T10)
                      n202 = global write "全局 时间2.vi" "平行样索引"(w213) -> ()
                    }
                  }
                }
                frame #3 {
                  n203 = call "数据处理整合 (子VI).vi"("枚举"=enum16{"实时数据排序", "小时数据排序"}."实时数据排序") -> ("已排序的数组"=w240:string[])  [unwired: 10 in]
                  n204 = Array Size(array=w240) -> (size(s)=w239:i32)
                  n205 = global write "全局 数据数组大小.vi" "数据数组大小"(w239) -> ()
                }
                frame #4 {
                  n206 = global read "全局 数据发送重叠.vi" "掉线指示灯"() -> (w241:bool)
                  n207 = case shown="False" w241 {
                    frame False {
                      n208 = global read "全局 数据数组大小.vi" "数据数组大小"() -> (w243:i32)
                      n209 = Greater Than 0?(x=w243) -> (x > 0?=w244:bool)
                      n210 = case shown="True" w244 {
                        tunnel: w243 -> [_ w245]
                        frame False {
                        }
                        frame True {
                          n211 = for {
                            N: w245 -> [_]
                            i -> [w248]
                            n212 = global write "全局 小时数据发送次数.vi" "小时数据发送次数"(w248) -> ()
                            n213 = Get Date/Time In Seconds() -> (seconds since 1Jan1904=w252:timestamp)
                            n214 = Format Date/Time String(time format string (%c)="%Y%m%d%H%M%S%3u" ("时间格式字符串(%c)"), seconds (now)=w252) -> (date/time string=w251:string)  [unwired: 1 in]
                            n215 = Search and Replace String(input string=w251, search string="." ("搜索字符串")) -> (result string=w249:string)  [unwired: 6 in, 3 out]
                            n216 = global read "断电保存全局.vi" "MN"() -> (w256:string)
                            n217 = global read "断电保存全局.vi" "PW"() -> (w255:string)
                            n218 = call "数据编码.vi"("table输入"="实时数据" ("新元素/子数组"), "QN"=w249, "MN"=w256, "PW"=w255) -> ("错误常量"=w254:errorcluster, "通讯包字符串"=w246:string)  [unwired: 10 in]
                            n219 = call "通信状态入队列.vi"("错误输入（无错误）"=w254, "发送报文"=w246, "枚举"=enum16{"打开连接", "发送数据", "读取数据", "数据处理", "关闭连接"}."发送数据") -> ()  [unwired: 8 in, 1 out]
                          }
                        }
                      }
                    }
                    frame True {
                    }
                  }
                }
              }
            }
            frame "集成干预" {
              n220 = flat-sequence {
                tunnel: [T1."集成干预"] -> w258
                frame #0 {
                  n221 = global write "全局 小时数据发送次数.vi" "小时数据发送次数"(0 ("小时数据发送次数")) -> ()
                  n222 = global write "全局1.vi" "枚举"(enum16{"返回请求应答", "上传数据", "返回执行结果"}."上传数据" ("枚举")) -> ()
                  n223 = global write "全局 实时数据参数.vi" "实时数据参数"("集成干预测试") -> ()
                }
                frame #1 {
                  (unwired) "f" ("列队名（唯一）")
                  n224 = call "从数据库获取数据通用可配置(子VI).vi"("table输入"="集成干预测试" ("新元素/子数组")) -> ()  [unwired: 9 in, 2 out]
                }
                frame #2 {
                  n225 = global read "全局 数据发送重叠.vi" "掉线指示灯"() -> (w265:bool)
                  n226 = Not(x=w265) -> (.not. x?=w264:bool)
                  n227 = case shown="True" w264 {
                    frame False {
                    }
                    frame True {
                      n228 = global read "全局 时间2.vi" "集成干预索引"() -> (w269:T12)
                      n229 = Cluster To Array(cluster=w269) -> (array=w268:string[])
                      n230 = for {
                        tunnel: [w271] -> w267 mode=indexing
                        tunnel: w268 -> [w270] mode=indexing
                        i -> [w272]
                        # "行数大于零"
                        n231 = case shown="17" w272 {
                          tunnel: [w277 w278 w279 w280 w281 w282 w283 w284 w285 w286 w287 w288 w289 w290 w291 w292 w293 w294] -> w273
                          frame 0, Default {
                            n232 = global read "全局 所有参数.vi" "氨氮"() -> (w277:string[][])
                          }
                          frame 1 {
                            n233 = global read "全局 所有参数.vi" "总磷"() -> (w278:string[][])
                          }
                          frame 2 {
                            n234 = global read "全局 所有参数.vi" "总氮"() -> (w279:string[][])
                          }
                          frame 3 {
                            n235 = global read "全局 所有参数.vi" "CODMn"() -> (w280:string[][])
                          }
                          frame 4 {
                            n236 = global read "全局 所有参数.vi" "CODCr"() -> (w281:string[][])
                          }
                          frame 5 {
                            n237 = global read "全局 所有参数.vi" "DO"() -> (w282:string[][])
                          }
                          frame 6 {
                            n238 = global read "全局 所有参数.vi" "PH"() -> (w283:string[][])
                          }
                          frame 7 {
                            n239 = global read "全局 所有参数.vi" "电导率"() -> (w284:string[][])
                          }
                          frame 8 {
                            n240 = global read "全局 所有参数.vi" "水温"() -> (w285:string[][])
                          }
                          frame 9 {
                            n241 = global read "全局 所有参数.vi" "浊度"() -> (w286:string[][])
                          }
                          frame 10 {
                            n242 = global read "全局 所有参数.vi" "叶绿素"() -> (w287:string[][])
                          }
                          frame 11 {
                            n243 = global read "全局 所有参数.vi" "藻密度"() -> (w288:string[][])
                          }
                          frame 12 {
                            n244 = global read "全局 所有参数.vi" "亚硝酸盐"() -> (w289:string[][])
                          }
                          frame 13 {
                            n245 = global read "全局 所有参数.vi" "硫化物"() -> (w290:string[][])
                          }
                          frame 14 {
                            n246 = global read "全局 所有参数.vi" "ORP"() -> (w291:string[][])
                          }
                          frame 15 {
                            n247 = global read "全局 所有参数.vi" "氟化物"() -> (w292:string[][])
                          }
                          frame 16 {
                            n248 = global read "全局 所有参数.vi" "挥发酚"() -> (w293:string[][])
                          }
                          frame 17 {
                            n249 = global read "全局 所有参数.vi" "氯化物"() -> (w294:string[][])
                          }
                        }
                        n250 = Array Size(array=w273) -> (size(s)=w275:i32[])
                        n251 = Index Array(array=w275) -> (element=w274:i32)  [unwired: 1 in]
                        n252 = Greater Than 0?(x=w274) -> (x > 0?=w276:bool)
                        n253 = case shown="True" w276 {
                          tunnel: w272 -> [_ _]
                          tunnel: w274 -> [_ _]
                          tunnel: w273 -> [_ w297]
                          tunnel: [w295 w296] -> w271
                          tunnel: w270 -> [w295 _]
                          frame False {
                          }
                          frame True {
                            # "最新时间戳加1分钟"
                            n254 = Array Size(array=w297) -> (size(s)=w301:i32[])
                            n255 = Index Array(array=w301) -> (element=w300:i32)  [unwired: 1 in]
                            n256 = Decrement(x=w300) -> (x-1=w299:i32)
                            n257 = Index Array(array=w297, index (row)=w299, index (col)=0 ("禁用的索引 (列)")) -> (element=w302:string)
                            n258 = call "日期时间字符串转换分钟数加一.vi"("data[0]"=w302) -> ("日期/时间字符串"=w296:string)  [unwired: 10 in]
                          }
                        }
                      }
                      n259 = Array To Cluster(array=w267) -> (cluster=w266:T13)
                      n260 = global write "全局 时间2.vi" "集成干预索引"(w266) -> ()
                    }
                  }
                }
                frame #3 {
                  n261 = call "数据处理整合 (子VI).vi"("枚举"=enum16{"实时数据排序", "小时数据排序"}."实时数据排序") -> ("已排序的数组"=w305:string[])  [unwired: 10 in]
                  n262 = Array Size(array=w305) -> (size(s)=w304:i32)
                  n263 = global write "全局 数据数组大小.vi" "数据数组大小"(w304) -> ()
                }
                frame #4 {
                  n264 = global read "全局 数据发送重叠.vi" "掉线指示灯"() -> (w307:bool)
                  n265 = case shown="False" w307 {
                    frame False {
                      n266 = global read "全局 数据数组大小.vi" "数据数组大小"() -> (w308:i32)
                      n267 = Greater Than 0?(x=w308) -> (x > 0?=w309:bool)
                      n268 = case shown="True" w309 {
                        tunnel: w308 -> [_ w310]
                        frame False {
                        }
                        frame True {
                          n269 = for {
                            N: w310 -> [_]
                            i -> [w313]
                            n270 = global write "全局 小时数据发送次数.vi" "小时数据发送次数"(w313) -> ()
                            n271 = Get Date/Time In Seconds() -> (seconds since 1Jan1904=w317:timestamp)
                            n272 = Format Date/Time String(time format string (%c)="%Y%m%d%H%M%S%3u" ("时间格式字符串(%c)"), seconds (now)=w317) -> (date/time string=w316:string)  [unwired: 1 in]
                            n273 = Search and Replace String(input string=w316, search string="." ("搜索字符串")) -> (result string=w314:string)  [unwired: 6 in, 3 out]
                            n274 = global read "断电保存全局.vi" "MN"() -> (w320:string)
                            n275 = global read "断电保存全局.vi" "PW"() -> (w319:string)
                            n276 = call "数据编码.vi"("table输入"="实时数据" ("新元素/子数组"), "QN"=w314, "MN"=w320, "PW"=w319) -> ("错误常量"=w321:errorcluster, "通讯包字符串"=w311:string)  [unwired: 10 in]
                            n277 = call "通信状态入队列.vi"("错误输入（无错误）"=w321, "发送报文"=w311, "枚举"=enum16{"打开连接", "发送数据", "读取数据", "数据处理", "关闭连接"}."发送数据") -> ()  [unwired: 8 in, 1 out]
                          }
                        }
                      }
                    }
                    frame True {
                    }
                  }
                }
              }
            }
          }
          n278 = Not(x=w25) -> (.not. x?=w26:bool)
          n279 = global write "全局1.vi" "核查数据上传"(w26) -> ()
        }
        n280 = global read "断电保存全局.vi" "日志、参数发送"() -> (w22:bool)
        n281 = case shown="False" w22 {
          tunnel: ["环境参数" ("组合框") "操作日志" ("组合框")] -> w23
          frame False {
          }
          frame True {
          }
        }
      }
      frame "操作日志" {
        # "间隔时间上传"
        # "直接1分钟查询 一次,有数据就按数据上传,没数据就不上传,在数据发送那边有做处理"
        n282 = flat-sequence {
          frame #0 {
            # "时间"
            n283 = call "日志信息主动发送(子VI).vi"() -> ()  [unwired: 12 in]
            n284 = global write "全局 小时数据发送次数.vi" "小时数据发送次数"(0 ("小时数据发送次数")) -> ()
            n285 = global write "全局1.vi" "枚举"(enum16{"返回请求应答", "上传数据", "返回执行结果"}."上传数据" ("枚举")) -> ()
          }
          frame #1 {
            n286 = call "获取操作日志 (子VI).vi"("table输入"="操作日志") -> ()  [unwired: 11 in]
          }
          frame #2 {
            n287 = call "数据处理整合 (子VI).vi"("枚举"=enum16{"实时数据排序", "小时数据排序"}."实时数据排序") -> ("已排序的数组"=w337:string[])  [unwired: 10 in]
            n288 = Array Size(array=w337) -> (size(s)=w336:i32)
            n289 = global write "全局 数据数组大小.vi" "数据数组大小"(w336) -> ()
          }
          frame #3 {
            n290 = global read "全局 数据发送重叠.vi" "掉线指示灯"() -> (w339:bool)
            n291 = Not(x=w339) -> (.not. x?=w338:bool)
            n292 = case shown="True" w338 {
              frame False {
              }
              frame True {
                n293 = global read "全局 时间2.vi" "仪器日志索引"() -> (w343:T14)
                n294 = Cluster To Array(cluster=w343) -> (array=w342:string[])
                n295 = for {
                  tunnel: w342 -> [w344] mode=indexing
                  tunnel: [w345] -> w340 mode=indexing
                  i -> [w347]
                  # "行数大于零"
                  n296 = case shown="7" w347 {
                    tunnel: [w351 w352 w353 w354 w355 w356 w357 w358] -> w346
                    frame 0, Default {
                      n297 = global read "全局 所有参数.vi" "氨氮"() -> (w351:string[][])
                    }
                    frame 1 {
                      n298 = global read "全局 所有参数.vi" "总磷"() -> (w352:string[][])
                    }
                    frame 2 {
                      n299 = global read "全局 所有参数.vi" "总氮"() -> (w353:string[][])
                    }
                    frame 3 {
                      n300 = global read "全局 所有参数.vi" "CODMn"() -> (w354:string[][])
                    }
                    frame 4 {
                      n301 = global read "全局 所有参数.vi" "CODCr"() -> (w355:string[][])
                    }
                    frame 5 {
                      n302 = global read "全局 所有参数.vi" "DO"() -> (w356:string[][])
                    }
                    frame 6 {
                      n303 = global read "全局 所有参数.vi" "氟化物"() -> (w357:string[][])
                    }
                    frame 7 {
                      n304 = global read "全局 所有参数.vi" "挥发酚"() -> (w358:string[][])
                    }
                  }
                  n305 = Array Size(array=w346) -> (size(s)=w349:i32[])
                  n306 = Index Array(array=w349) -> (element=w348:i32)  [unwired: 1 in]
                  n307 = Greater Than 0?(x=w348) -> (x > 0?=w350:bool)
                  n308 = case shown="True" w350 {
                    tunnel: w348 -> [_ _]
                    tunnel: w346 -> [_ w364]
                    tunnel: [w359 w360] -> w345
                    tunnel: w344 -> [w359 _]
                    frame False {
                    }
                    frame True {
                      # "最新时间戳加1分钟"
                      n309 = Array Size(array=w364) -> (size(s)=w366:i32[])
                      n310 = Index Array(array=w366) -> (element=w365:i32)  [unwired: 1 in]
                      n311 = Decrement(x=w365) -> (x-1=w363:i32)
                      n312 = Index Array(array=w364, index (row)=w363, index (col)=0 ("禁用的索引 (列)")) -> (element=w361:string)
                      n313 = call "日期时间字符串转换秒数加一.vi"("data[0]"=w361) -> ("日期/时间字符串"=w360:string)  [unwired: 10 in]
                    }
                  }
                }
                n314 = Array To Cluster(array=w340) -> (cluster=w341:T15)
                n315 = global write "全局 时间2.vi" "仪器日志索引"(w341) -> ()
              }
            }
          }
          frame #4 {
            # "判定是否存表"
            n316 = global read "全局 数据发送重叠.vi" "掉线指示灯"() -> (w367:bool)
            n317 = case shown="False" w367 {
              frame False {
                n318 = global read "全局 数据数组大小.vi" "数据数组大小"() -> (w368:i32)
                n319 = Greater Than 0?(x=w368) -> (x > 0?=w369:bool)
                n320 = case shown="True" w369 {
                  frame False {
                  }
                  frame True {
                    n321 = while {
                      stop <- w370 stop-if-true
                      n322 = global read "全局 数据数组大小.vi" "数据数组大小"() -> (w374:i32)
                      n323 = global read "全局 小时数据发送次数.vi" "小时数据发送次数"() -> (w373:i32)
                      n324 = Decrement(x=w374) -> (x-1=w375:i32)
                      n325 = Greater Or Equal?(x=w373, y=w375) -> (x >= y?=w370:bool)
                      n326 = Get Date/Time In Seconds() -> (seconds since 1Jan1904=w382:timestamp)
                      n327 = Format Date/Time String(time format string (%c)="%Y%m%d%H%M%S%3u" ("时间格式字符串(%c)"), seconds (now)=w382) -> (date/time string=w381:string)  [unwired: 1 in]
                      n328 = Search and Replace String(input string=w381, search string="." ("搜索字符串")) -> (result string=w379:string)  [unwired: 6 in, 3 out]
                      n329 = global read "断电保存全局.vi" "MN"() -> (w378:string)
                      n330 = global read "断电保存全局.vi" "PW"() -> (w377:string)
                      n331 = call "数据编码.vi"("table输入"="操作日志" ("新元素/子数组"), "QN"=w379, "MN"=w378, "PW"=w377) -> ("错误常量"=w376:errorcluster, "通讯包字符串"=w371:string)  [unwired: 10 in]
                      n332 = call "通信状态入队列.vi"("错误输入（无错误）"=w376, "发送报文"=w371, "枚举"=enum16{"打开连接", "发送数据", "读取数据", "数据处理", "关闭连接"}."发送数据") -> ()  [unwired: 8 in, 1 out]
                    }
                  }
                }
              }
              frame True {
              }
            }
          }
        }
        n333 = global read "断电保存全局.vi" "应用环境"() -> (w329:T2)
        n334 = case shown="\"GB212\", Default" w329 {
          tunnel: ["3092日志信息" ("组合框") "系统状态" ("组合框")] -> w328
          frame "STD" {
          }
          frame "GB212", Default {
          }
        }
      }
      frame "3092日志信息" {
        # "间隔时间上传"
        # "直接1分钟查询 一次,有数据就按数据上传,没数据就不上传,在数据发送那边有做处理"
        n335 = flat-sequence {
          tunnel: [w390] -> w386
          tunnel: w386 -> [w394]
          frame #0 {
            n336 = global write "全局 小时数据发送次数.vi" "小时数据发送次数"(0 ("小时数据发送次数")) -> ()
            n337 = global write "全局1.vi" "枚举"(enum16{"返回请求应答", "上传数据", "返回执行结果"}."上传数据" ("枚举")) -> ()
          }
          frame #1 {
            n338 = call "数据表比对.vi"("table输入"="3092日志信息") -> ("待发送数据"=w390:string[][])  [unwired: 7 in, 3 out]
            n339 = global write "全局 所有参数.vi" "CODMn"(w390) -> ()
          }
          frame #2 {
            n340 = Array Size(array=w394) -> (size(s)=w393:i32[])
            n341 = Index Array(array=w393) -> (element=w392:i32)  [unwired: 1 in]
            n342 = global write "全局 数据数组大小.vi" "数据数组大小"(w392) -> ()
          }
          frame #3 {
            n343 = global read "全局 数据发送重叠.vi" "掉线指示灯"() -> (w396:bool)
            n344 = Not(x=w396) -> (.not. x?=w395:bool)
            n345 = case shown="True" w395 {
              frame False {
              }
              frame True {
                # "行数大于零"
                n346 = global read "全局 所有参数.vi" "CODMn"() -> (w399:string[][])
                n347 = global read "全局 时间2.vi" "3092日志索引起始时间"() -> (w398:string)
                n348 = Array Size(array=w399) -> (size(s)=w401:i32[])
                n349 = Index Array(array=w401) -> (element=w400:i32)  [unwired: 1 in]
                n350 = Greater Than 0?(x=w400) -> (x > 0?=w402:bool)
                n351 = case shown="True" w402 {
                  tunnel: w400 -> [_ _]
                  tunnel: w399 -> [_ w408]
                  tunnel: [w403 w404] -> w397
                  tunnel: w398 -> [w403 _]
                  frame False {
                  }
                  frame True {
                    # "最新时间戳加1分钟"
                    n352 = Array Size(array=w408) -> (size(s)=w410:i32[])
                    n353 = Index Array(array=w410) -> (element=w409:i32)  [unwired: 1 in]
                    n354 = Decrement(x=w409) -> (x-1=w407:i32)
                    n355 = Index Array(array=w408, index (row)=w407, index (col)=0 ("禁用的索引 (列)")) -> (element=w405:string)
                    n356 = call "日期时间字符串转换秒数加一.vi"("data[0]"=w405) -> ("日期/时间字符串"=w404:string)  [unwired: 10 in]
                  }
                }
                n357 = global write "全局 时间2.vi" "3092日志索引起始时间"(w397) -> ()
              }
            }
          }
          frame #4 {
            # "判定是否存表"
            n358 = global read "全局 数据发送重叠.vi" "掉线指示灯"() -> (w411:bool)
            n359 = case shown="False" w411 {
              frame False {
                n360 = global read "全局 数据数组大小.vi" "数据数组大小"() -> (w412:i32)
                n361 = Greater Than 0?(x=w412) -> (x > 0?=w413:bool)
                n362 = case shown="True" w413 {
                  frame False {
                  }
                  frame True {
                    n363 = while {
                      stop <- w416 stop-if-true
                      n364 = global read "全局 数据数组大小.vi" "数据数组大小"() -> (w418:i32)
                      n365 = global read "全局 小时数据发送次数.vi" "小时数据发送次数"() -> (w417:i32)
                      n366 = Decrement(x=w418) -> (x-1=w419:i32)
                      n367 = Greater Or Equal?(x=w417, y=w419) -> (x >= y?=w416:bool)
                      n368 = Get Date/Time In Seconds() -> (seconds since 1Jan1904=w426:timestamp)
                      n369 = Format Date/Time String(time format string (%c)="%Y%m%d%H%M%S%3u" ("时间格式字符串(%c)"), seconds (now)=w426) -> (date/time string=w425:string)  [unwired: 1 in]
                      n370 = Search and Replace String(input string=w425, search string="." ("搜索字符串")) -> (result string=w423:string)  [unwired: 6 in, 3 out]
                      n371 = global read "断电保存全局.vi" "MN"() -> (w422:string)
                      n372 = global read "断电保存全局.vi" "PW"() -> (w421:string)
                      n373 = call "数据编码.vi"("table输入"="3092日志信息" ("新元素/子数组"), "QN"=w423, "MN"=w422, "PW"=w421) -> ("错误常量"=w420:errorcluster, "通讯包字符串"=w414:string)  [unwired: 10 in]
                      n374 = call "通信状态入队列.vi"("错误输入（无错误）"=w420, "发送报文"=w414, "枚举"=enum16{"打开连接", "发送数据", "读取数据", "数据处理", "关闭连接"}."发送数据") -> ()  [unwired: 8 in, 1 out]
                    }
                  }
                }
              }
              frame True {
              }
            }
          }
        }
      }
      frame "系统状态" {
        # "直接1分钟查询 一次,有变化就按上传,没变化就不上传"
        n375 = flat-sequence {
          frame #0 {
            # "时间"
            n376 = global write "全局 小时数据发送次数.vi" "小时数据发送次数"(0 ("小时数据发送次数")) -> ()
            n377 = global write "全局 数据数组大小.vi" "数据数组大小"(1 ("数据数组大小")) -> ()
            n378 = global write "全局1.vi" "枚举"(enum16{"返回请求应答", "上传数据", "返回执行结果"}."上传数据" ("枚举")) -> ()
          }
          frame #1 {
            # "判定是否存表"
            n379 = global read "全局 数据发送重叠.vi" "掉线指示灯"() -> (w438:bool)
            n380 = case shown="False" w438 {
              frame False {
                n381 = global read "全局1.vi" "系统状态"() -> (w439:bool)
                n382 = case shown="True" w439 {
                  frame False {
                  }
                  frame True {
                    n383 = global write "全局1.vi" "系统状态"(FALSE ("系统状态")) -> ()
                    n384 = for {
                      N: 6 -> [_]
                      n385 = flat-sequence {
                        frame #0 {
                          n386 = Get Date/Time In Seconds() -> (seconds since 1Jan1904=w450:timestamp)
                          n387 = Format Date/Time String(time format string (%c)="%Y%m%d%H%M%S%3u" ("时间格式字符串(%c)"), seconds (now)=w450) -> (date/time string=w449:string)  [unwired: 1 in]
                          n388 = Search and Replace String(input string=w449, search string="." ("搜索字符串")) -> (result string=w447:string)  [unwired: 6 in, 3 out]
                          n389 = global read "断电保存全局.vi" "MN"() -> (w446:string)
                          n390 = global read "断电保存全局.vi" "PW"() -> (w445:string)
                          n391 = call "数据编码.vi"("table输入"="系统状态" ("新元素/子数组"), "QN"=w447, "MN"=w446, "PW"=w445) -> ("错误常量"=w444:errorcluster, "通讯包字符串"=w442:string)  [unwired: 10 in]
                          n392 = call "通信状态入队列.vi"("错误输入（无错误）"=w444, "发送报文"=w442, "枚举"=enum16{"打开连接", "发送数据", "读取数据", "数据处理", "关闭连接"}."发送数据") -> ()  [unwired: 8 in, 1 out]
                        }
                        frame #1 {
                          n393 = global read "全局 小时数据发送次数.vi" "小时数据发送次数"() -> (w454:i32)
                          n394 = Increment(x=w454) -> (x+1=w453:i32)
                          n395 = global write "全局 小时数据发送次数.vi" "小时数据发送次数"(w453) -> ()
                        }
                      }
                    }
                  }
                }
              }
              frame True {
              }
            }
          }
        }
        n396 = global read "断电保存全局.vi" "应用环境"() -> (w430:T2)
        n397 = case shown="\"GB212\", Default" w430 {
          tunnel: ["运行模式" ("组合框") "超标留样" ("组合框")] -> w431
          frame "STD" {
            n398 = global write "全局 数据发送重叠.vi" "数据接收超时指示灯"(FALSE ("数据接收超时指示灯")) -> ()
          }
          frame "GB212", Default {
          }
        }
      }
      frame "运行模式" {
        # "直接1分钟查询 一次,有变化就按上传,没变化就不上传"
        n399 = flat-sequence {
          frame #0 {
            # "时间"
            n400 = global write "全局 小时数据发送次数.vi" "小时数据发送次数"(0 ("小时数据发送次数")) -> ()
            n401 = global write "全局 数据数组大小.vi" "数据数组大小"(1 ("数据数组大小")) -> ()
            n402 = global write "全局1.vi" "枚举"(enum16{"返回请求应答", "上传数据", "返回执行结果"}."上传数据" ("枚举")) -> ()
          }
          frame #1 {
            # "判定是否存表"
            n403 = global read "全局 数据发送重叠.vi" "掉线指示灯"() -> (w460:bool)
            n404 = case shown="False" w460 {
              frame False {
                n405 = global read "全局1.vi" "运行模式"() -> (w461:bool)
                n406 = case shown="True" w461 {
                  frame False {
                  }
                  frame True {
                    n407 = global read "全局 小时数据发送次数.vi" "小时数据发送次数"() -> (w472:i32)
                    n408 = global write "全局1.vi" "运行模式"(FALSE ("系统状态")) -> ()
                    n409 = Increment(x=w472) -> (x+1=w471:i32)
                    n410 = global write "全局 小时数据发送次数.vi" "小时数据发送次数"(w471) -> ()
                    n411 = Get Date/Time In Seconds() -> (seconds since 1Jan1904=w475:timestamp)
                    n412 = Format Date/Time String(time format string (%c)="%Y%m%d%H%M%S%3u" ("时间格式字符串(%c)"), seconds (now)=w475) -> (date/time string=w474:string)  [unwired: 1 in]
                    n413 = Search and Replace String(input string=w474, search string="." ("搜索字符串")) -> (result string=w466:string)  [unwired: 6 in, 3 out]
                    n414 = global read "断电保存全局.vi" "MN"() -> (w470:string)
                    n415 = global read "断电保存全局.vi" "PW"() -> (w469:string)
                    n416 = call "数据编码.vi"("table输入"="运行模式" ("新元素/子数组"), "QN"=w466, "MN"=w470, "PW"=w469) -> ("错误常量"=w468:errorcluster, "通讯包字符串"=w462:string)  [unwired: 10 in]
                    n417 = global read "断电保存全局.vi" "应用环境"() -> (w464:T2)
                    n418 = call "通信状态入队列.vi"("错误输入（无错误）"=w468, "发送报文"=w462, "枚举"=enum16{"打开连接", "发送数据", "读取数据", "数据处理", "关闭连接"}."发送数据") -> ("错误输出"=w465:errorcluster)  [unwired: 8 in]
                    n419 = case shown="\"STD\"" w464 {
                      tunnel: w466 -> [w481 _]
                      tunnel: w462 -> [w480 _]
                      tunnel: w465 -> [w479 _]
                      frame "STD" {
                        n420 = global read "断电保存全局.vi" "判断数据反馈"() -> (w478:enum16{"非严格判断", "严格判断", "不判断"})
                        n421 = case shown="\"严格判断\"" w478 {
                          tunnel: w480 -> [_ w486]
                          tunnel: w479 -> [_ w485]
                          tunnel: w481 -> [_ w484]
                          frame "不判断", Default {
                          }
                          frame "严格判断" {
                            n422 = global read "断电保存全局.vi" "数据发送通道"() -> (w483:enum16{"TCP", "VISA"})
                            n423 = call "数据补发判定有限循环.vi"("错误输入（无错误）"=w485, "数据输入"=w486, "QN"=w484, "数据发送通道"=w483) -> ("error out"=w482:errorcluster)  [unwired: 7 in]
                            n424 = case shown="No Error" w482 {
                              frame No Error {
                                n425 = global read "全局 数据发送重叠.vi" "数据接收超时指示灯"() -> (w487:bool)
                                n426 = case shown="True" w487 {
                                frame False {
                                }
                                frame True {
                                n427 = global write "全局1.vi" "测量周期"(TRUE ("测量周期")) -> ()
                                }
                                }
                              }
                              frame Error {
                              }
                            }
                          }
                        }
                      }
                      frame "GB212", Default {
                      }
                    }
                  }
                }
              }
              frame True {
              }
            }
          }
        }
      }
      frame "测量周期" {
        # "直接1分钟查询 一次,有变化就按上传,没变化就不上传"
        n428 = flat-sequence {
          frame #0 {
            # "时间"
            n429 = global write "全局 小时数据发送次数.vi" "小时数据发送次数"(0 ("小时数据发送次数")) -> ()
            n430 = global write "全局1.vi" "枚举"(enum16{"返回请求应答", "上传数据", "返回执行结果"}."上传数据" ("枚举")) -> ()
            n431 = global write "全局 数据数组大小.vi" "数据数组大小"(1 ("数据数组大小")) -> ()
          }
          frame #1 {
            # "判定是否存表"
            n432 = global read "全局 数据发送重叠.vi" "掉线指示灯"() -> (w494:bool)
            n433 = case shown="False" w494 {
              frame False {
                n434 = global read "全局1.vi" "测量周期"() -> (w495:bool)
                n435 = case shown="True" w495 {
                  frame False {
                  }
                  frame True {
                    n436 = global read "全局1.vi" "读取各参数测量周期的值"() -> (w503:u16[])
                    n437 = global write "全局1.vi" "测量周期"(FALSE ("系统状态")) -> ()
                    n438 = for {
                      tunnel: w503 -> [w548] mode=indexing
                      shift-right: [w546] -> w507
                      shift-left: u16[] [] ("读取各参数测量周期的值") -> [w549]
                      n439 = Not Equal To 0?(x=w548) -> (x != 0?=w547:bool)
                      n440 = case shown="True" w547 {
                        tunnel: w549 -> [w550 w553]
                        tunnel: w548 -> [_ w552]
                        tunnel: [w550 w551] -> w546
                        frame False {
                        }
                        frame True {
                          n441 = Insert Into Array(array=w553, new element=w552) -> (w551:u16[])  [unwired: 1 in]
                        }
                      }
                    }
                    n442 = global read "断电保存全局.vi" "应用环境"() -> (w501:T2)
                    n443 = Array Max & Min(array=w507) -> (max value=w506:u16, min value=w505:u16)  [unwired: 2 out]
                    n444 = Not Equal?(x=w506, y=w505) -> (x != y?=w508:bool)
                    n445 = Equal?(x=w501, y=应用环境."STD") -> (x = y?=w502:bool)
                    n446 = And(x=w508, y=w502) -> (x .and. y?=w509:bool)
                    n447 = case shown="True" w509 {
                      tunnel: [w525 w537] -> w499
                      tunnel: [w524 w536] -> w498
                      tunnel: [w522 w534] -> w497
                      frame False {
                        n448 = Get Date/Time In Seconds() -> (seconds since 1Jan1904=w531:timestamp)
                        n449 = Format Date/Time String(time format string (%c)="%Y%m%d%H%M%S%3u" ("时间格式字符串(%c)"), seconds (now)=w531) -> (date/time string=w530:string)  [unwired: 1 in]
                        n450 = Search and Replace String(input string=w530, search string="." ("搜索字符串")) -> (result string=w524:string)  [unwired: 6 in, 3 out]
                        n451 = global read "断电保存全局.vi" "MN"() -> (w528:string)
                        n452 = global read "断电保存全局.vi" "PW"() -> (w527:string)
                        n453 = call "数据编码.vi"("table输入"="测量周期" ("新元素/子数组"), "QN"=w524, "MN"=w528, "PW"=w527) -> ("错误常量"=w526:errorcluster, "通讯包字符串"=w522:string)  [unwired: 10 in]
                        n454 = call "通信状态入队列.vi"("错误输入（无错误）"=w526, "发送报文"=w522, "枚举"=enum16{"打开连接", "发送数据", "读取数据", "数据处理", "关闭连接"}."发送数据") -> ("错误输出"=w525:errorcluster)  [unwired: 8 in]
                      }
                      frame True {
                        # "STD&参数测量周期不一样"
                        n455 = Get Date/Time In Seconds() -> (seconds since 1Jan1904=w543:timestamp)
                        n456 = Format Date/Time String(time format string (%c)="%Y%m%d%H%M%S%3u" ("时间格式字符串(%c)"), seconds (now)=w543) -> (date/time string=w542:string)  [unwired: 1 in]
                        n457 = Search and Replace String(input string=w542, search string="." ("搜索字符串")) -> (result string=w536:string)  [unwired: 6 in, 3 out]
                        n458 = global read "断电保存全局.vi" "MN"() -> (w540:string)
                        n459 = global read "断电保存全局.vi" "PW"() -> (w539:string)
                        n460 = call "数据编码.vi"("table输入"="各参数测量周期" ("新元素/子数组"), "QN"=w536, "MN"=w540, "PW"=w539) -> ("错误常量"=w538:errorcluster, "通讯包字符串"=w534:string)  [unwired: 10 in]
                        n461 = call "通信状态入队列.vi"("错误输入（无错误）"=w538, "发送报文"=w534, "枚举"=enum16{"打开连接", "发送数据", "读取数据", "数据处理", "关闭连接"}."发送数据") -> ("错误输出"=w537:errorcluster)  [unwired: 8 in]
                      }
                    }
                    n462 = global read "断电保存全局.vi" "应用环境"() -> (w500:T2)
                    n463 = case shown="\"STD\"" w500 {
                      tunnel: w498 -> [w514 _]
                      tunnel: w497 -> [w513 _]
                      tunnel: w499 -> [w512 _]
                      frame "STD" {
                        n464 = global read "断电保存全局.vi" "判断数据反馈"() -> (w511:enum16{"非严格判断", "严格判断", "不判断"})
                        n465 = case shown="\"严格判断\"" w511 {
                          tunnel: w513 -> [_ w519]
                          tunnel: w512 -> [_ w518]
                          tunnel: w514 -> [_ w517]
                          frame "不判断", Default {
                          }
                          frame "严格判断" {
                            n466 = global read "断电保存全局.vi" "数据发送通道"() -> (w516:enum16{"TCP", "VISA"})
                            n467 = call "数据补发判定有限循环.vi"("错误输入（无错误）"=w518, "数据输入"=w519, "QN"=w517, "数据发送通道"=w516) -> ("error out"=w515:errorcluster)  [unwired: 7 in]
                            n468 = case shown="No Error" w515 {
                              frame No Error {
                                n469 = global read "全局 数据发送重叠.vi" "数据接收超时指示灯"() -> (w520:bool)
                                n470 = case shown="True" w520 {
                                frame False {
                                }
                                frame True {
                                n471 = global write "全局1.vi" "测量周期"(TRUE ("测量周期")) -> ()
                                }
                                }
                              }
                              frame Error {
                              }
                            }
                          }
                        }
                      }
                      frame "GB212", Default {
                      }
                    }
                  }
                }
              }
              frame True {
              }
            }
          }
        }
      }
      frame "超标留样" {
        # "直接1分钟查询 一次,有变化就按上传,没变化就不上传"
        n472 = flat-sequence {
          frame #0 {
            # "时间"
            n473 = global write "全局 小时数据发送次数.vi" "小时数据发送次数"(0 ("小时数据发送次数")) -> ()
            n474 = global write "全局 数据数组大小.vi" "数据数组大小"(1 ("数据数组大小")) -> ()
            n475 = global write "全局1.vi" "枚举"(enum16{"返回请求应答", "上传数据", "返回执行结果"}."上传数据" ("枚举")) -> ()
          }
          frame #1 {
            # "判定是否存表"
            n476 = global read "全局 数据发送重叠.vi" "掉线指示灯"() -> (w559:bool)
            n477 = case shown="False" w559 {
              frame False {
                n478 = global read "全局1.vi" "超标留样"() -> (w560:bool)
                n479 = case shown="True" w560 {
                  frame False {
                  }
                  frame True {
                    n480 = global read "全局 小时数据发送次数.vi" "小时数据发送次数"() -> (w568:i32)
                    n481 = global write "全局1.vi" "超标留样"(FALSE ("系统状态")) -> ()
                    n482 = Increment(x=w568) -> (x+1=w567:i32)
                    n483 = Get Date/Time In Seconds() -> (seconds since 1Jan1904=w572:timestamp)
                    n484 = global write "全局 小时数据发送次数.vi" "小时数据发送次数"(w567) -> ()
                    n485 = Format Date/Time String(time format string (%c)="%Y%m%d%H%M%S%3u" ("时间格式字符串(%c)"), seconds (now)=w572) -> (date/time string=w571:string)  [unwired: 1 in]
                    n486 = global read "断电保存全局.vi" "MN"() -> (w565:string)
                    n487 = global read "断电保存全局.vi" "PW"() -> (w564:string)
                    n488 = Search and Replace String(input string=w571, search string="." ("搜索字符串")) -> (result string=w569:string)  [unwired: 6 in, 3 out]
                    n489 = call "数据编码.vi"("table输入"="超标留样" ("新元素/子数组"), "QN"=w569, "MN"=w565, "PW"=w564) -> ("错误常量"=w566:errorcluster, "通讯包字符串"=w561:string)  [unwired: 10 in]
                    n490 = call "通信状态入队列.vi"("错误输入（无错误）"=w566, "发送报文"=w561, "枚举"=enum16{"打开连接", "发送数据", "读取数据", "数据处理", "关闭连接"}."发送数据") -> ()  [unwired: 8 in, 1 out]
                  }
                }
              }
              frame True {
              }
            }
          }
        }
      }
      frame "报警信息" {
        # "间隔时间上传"
        # "直接1分钟查询 一次,有数据就按数据上传,没数据为空的不传,在数据发送那边有做处理"
        n491 = flat-sequence {
          frame #0 {
            n492 = call "变量初始化.vi"() -> ()  [unwired: 11 in, 1 out]
          }
          frame #1 {
            # "分钟时间间隔"
            n493 = call "日志信息主动发送(子VI).vi"() -> ()  [unwired: 12 in]
            n494 = global write "全局 小时数据发送次数.vi" "小时数据发送次数"(0 ("小时数据发送次数")) -> ()
            n495 = global write "全局1.vi" "枚举"(enum16{"返回请求应答", "上传数据", "返回执行结果"}."上传数据" ("枚举")) -> ()
          }
          frame #2 {
            n496 = call "获取报警信息 (子VI).vi"() -> ()  [unwired: 12 in]
          }
          frame #3 {
            n497 = call "数据处理整合 (子VI).vi"("枚举"=enum16{"实时数据排序", "小时数据排序"}."实时数据排序") -> ("已排序的数组"=w587:string[])  [unwired: 10 in]
            n498 = Array Size(array=w587) -> (size(s)=w586:i32)
            n499 = global write "全局 数据数组大小.vi" "数据数组大小"(w586) -> ()
          }
          frame #4 {
            n500 = global read "全局 数据发送重叠.vi" "掉线指示灯"() -> (w589:bool)
            n501 = Not(x=w589) -> (.not. x?=w588:bool)
            n502 = case shown="True" w588 {
              frame False {
              }
              frame True {
                n503 = global read "全局 时间2.vi" "报警信息索引"() -> (w593:T16)
                n504 = Cluster To Array(cluster=w593) -> (array=w592:string[])
                n505 = for {
                  tunnel: [w595] -> w590 mode=indexing
                  tunnel: w592 -> [w594] mode=indexing
                  i -> [w597]
                  # "行数大于零"
                  n506 = case shown="13" w597 {
                    tunnel: [w601 w602 w603 w604 w605 w606 w607 w608 w609 w610 w611 w612 w613 w614] -> w596
                    frame 0, Default {
                      n507 = global read "全局 所有参数.vi" "氨氮"() -> (w601:string[][])
                    }
                    frame 1 {
                      n508 = global read "全局 所有参数.vi" "总磷"() -> (w602:string[][])
                    }
                    frame 2 {
                      n509 = global read "全局 所有参数.vi" "总氮"() -> (w603:string[][])
                    }
                    frame 3 {
                      n510 = global read "全局 所有参数.vi" "CODMn"() -> (w604:string[][])
                    }
                    frame 4 {
                      n511 = global read "全局 所有参数.vi" "CODCr"() -> (w605:string[][])
                    }
                    frame 5 {
                      n512 = global read "全局 所有参数.vi" "DO"() -> (w606:string[][])
                    }
                    frame 6 {
                      n513 = global read "全局 所有参数.vi" "PH"() -> (w607:string[][])
                    }
                    frame 7 {
                      n514 = global read "全局 所有参数.vi" "电导率"() -> (w608:string[][])
                    }
                    frame 8 {
                      n515 = global read "全局 所有参数.vi" "水温"() -> (w609:string[][])
                    }
                    frame 9 {
                      n516 = global read "全局 所有参数.vi" "浊度"() -> (w610:string[][])
                    }
                    frame 10 {
                      n517 = global read "全局 所有参数.vi" "叶绿素"() -> (w611:string[][])
                    }
                    frame 11 {
                      n518 = global read "全局 所有参数.vi" "藻密度"() -> (w612:string[][])
                    }
                    frame 12 {
                      n519 = global read "全局 所有参数.vi" "氟化物"() -> (w613:string[][])
                    }
                    frame 13 {
                      n520 = global read "全局 所有参数.vi" "挥发酚"() -> (w614:string[][])
                    }
                  }
                  n521 = Array Size(array=w596) -> (size(s)=w599:i32[])
                  n522 = Index Array(array=w599) -> (element=w598:i32)  [unwired: 1 in]
                  n523 = Greater Than 0?(x=w598) -> (x > 0?=w600:bool)
                  n524 = case shown="True" w600 {
                    tunnel: w598 -> [_ _]
                    tunnel: w596 -> [_ w619]
                    tunnel: [w615 w616] -> w595
                    tunnel: w594 -> [w615 _]
                    frame False {
                    }
                    frame True {
                      # "最新时间戳加1分钟"
                      n525 = Array Size(array=w619) -> (size(s)=w621:i32[])
                      n526 = Index Array(array=w621) -> (element=w620:i32)  [unwired: 1 in]
                      n527 = Decrement(x=w620) -> (x-1=w618:i32)
                      n528 = Index Array(array=w619, index (row)=w618, index (col)=0 ("禁用的索引 (列)")) -> (element=w622:string)
                      n529 = call "日期时间字符串转换分钟数加一.vi"("data[0]"=w622) -> ("日期/时间字符串"=w616:string)  [unwired: 10 in]
                    }
                  }
                }
                n530 = Array To Cluster(array=w590) -> (cluster=w591:T17)
                n531 = global write "全局 时间2.vi" "报警信息索引"(w591) -> ()
              }
            }
          }
          frame #5 {
            # "判定是否存表"
            n532 = global read "全局 数据发送重叠.vi" "掉线指示灯"() -> (w623:bool)
            n533 = case shown="False" w623 {
              frame False {
                # "判定数据不为空才发"
                n534 = global read "全局 数据数组大小.vi" "数据数组大小"() -> (w624:i32)
                n535 = Greater Than 0?(x=w624) -> (x > 0?=w625:bool)
                n536 = case shown="True" w625 {
                  frame False {
                    n537 = global write "全局1.vi" "核查数据上传"(FALSE ("数据上传")) -> ()
                  }
                  frame True {
                    n538 = while {
                      stop <- w629 stop-if-true
                      n539 = global read "全局 数据数组大小.vi" "数据数组大小"() -> (w631:i32)
                      n540 = global read "全局 小时数据发送次数.vi" "小时数据发送次数"() -> (w632:i32)
                      n541 = Decrement(x=w631) -> (x-1=w630:i32)
                      n542 = Greater Or Equal?(x=w632, y=w630) -> (x >= y?=w629:bool)
                      n543 = Get Date/Time In Seconds() -> (seconds since 1Jan1904=w639:timestamp)
                      n544 = Format Date/Time String(time format string (%c)="%Y%m%d%H%M%S%3u" ("时间格式字符串(%c)"), seconds (now)=w639) -> (date/time string=w638:string)  [unwired: 1 in]
                      n545 = Search and Replace String(input string=w638, search string="." ("搜索字符串")) -> (result string=w636:string)  [unwired: 6 in, 3 out]
                      n546 = global read "断电保存全局.vi" "MN"() -> (w635:string)
                      n547 = global read "断电保存全局.vi" "PW"() -> (w634:string)
                      n548 = call "数据编码.vi"("table输入"="报警信息" ("新元素/子数组"), "QN"=w636, "MN"=w635, "PW"=w634) -> ("错误常量"=w633:errorcluster, "通讯包字符串"=w627:string)  [unwired: 10 in]
                      n549 = call "通信状态入队列.vi"("错误输入（无错误）"=w633, "发送报文"=w627, "枚举"=enum16{"打开连接", "发送数据", "读取数据", "数据处理", "关闭连接"}."发送数据") -> ()  [unwired: 8 in, 1 out]
                    }
                  }
                }
              }
              frame True {
              }
            }
          }
        }
        n550 = global read "断电保存全局.vi" "应用环境"() -> (w577:T2)
        n551 = case shown="\"GB212\", Default" w577 {
          tunnel: ["3093报警信息" ("组合框") w580] -> w576
          frame "STD" {
          }
          frame "GB212", Default {
            n552 = global read "断电保存全局.vi" "仪器参数发送"() -> (w579:bool)
            n553 = case shown="True" w579 {
              tunnel: ["环境参数" ("组合框") "仪器参数" ("组合框")] -> w580
              frame False {
              }
              frame True {
              }
            }
          }
        }
      }
      frame "3093报警信息" {
        # "间隔时间上传"
        # "直接1分钟查询 一次,有数据就按数据上传,没数据为空的不传,在数据发送那边有做处理"
        n554 = flat-sequence {
          tunnel: [w650] -> w645
          tunnel: w645 -> [w654]
          frame #0 {
            n555 = global write "全局 小时数据发送次数.vi" "小时数据发送次数"(0 ("小时数据发送次数")) -> ()
            n556 = global write "全局1.vi" "枚举"(enum16{"返回请求应答", "上传数据", "返回执行结果"}."上传数据" ("枚举")) -> ()
          }
          frame #1 {
            n557 = call "数据表比对.vi"("table输入"="3093报警信息") -> ("待发送数据"=w650:string[][])  [unwired: 7 in, 3 out]
            n558 = global write "全局 所有参数.vi" "CODMn"(w650) -> ()
          }
          frame #2 {
            n559 = Array Size(array=w654) -> (size(s)=w653:i32[])
            n560 = Index Array(array=w653) -> (element=w652:i32)  [unwired: 1 in]
            n561 = global write "全局 数据数组大小.vi" "数据数组大小"(w652) -> ()
          }
          frame #3 {
            n562 = global read "全局 数据发送重叠.vi" "掉线指示灯"() -> (w656:bool)
            n563 = Not(x=w656) -> (.not. x?=w655:bool)
            n564 = case shown="True" w655 {
              frame False {
              }
              frame True {
                # "行数大于零"
                n565 = global read "全局 所有参数.vi" "CODMn"() -> (w659:string[][])
                n566 = global read "全局 时间2.vi" "3093报警索引起始时间"() -> (w658:string)
                n567 = Array Size(array=w659) -> (size(s)=w661:i32[])
                n568 = Index Array(array=w661) -> (element=w660:i32)  [unwired: 1 in]
                n569 = Greater Than 0?(x=w660) -> (x > 0?=w662:bool)
                n570 = case shown="True" w662 {
                  tunnel: w660 -> [_ _]
                  tunnel: w659 -> [_ w668]
                  tunnel: [w663 w664] -> w657
                  tunnel: w658 -> [w663 _]
                  frame False {
                  }
                  frame True {
                    # "最新时间戳加1分钟"
                    n571 = Array Size(array=w668) -> (size(s)=w670:i32[])
                    n572 = Index Array(array=w670) -> (element=w669:i32)  [unwired: 1 in]
                    n573 = Decrement(x=w669) -> (x-1=w667:i32)
                    n574 = Index Array(array=w668, index (row)=w667, index (col)=0 ("禁用的索引 (列)")) -> (element=w665:string)
                    n575 = call "日期时间字符串转换秒数加一.vi"("data[0]"=w665) -> ("日期/时间字符串"=w664:string)  [unwired: 10 in]
                  }
                }
                n576 = global write "全局 时间2.vi" "3093报警索引起始时间"(w657) -> ()
              }
            }
          }
          frame #4 {
            # "判定是否存表"
            n577 = global read "全局 数据发送重叠.vi" "掉线指示灯"() -> (w671:bool)
            n578 = case shown="False" w671 {
              frame False {
                n579 = global read "全局 数据数组大小.vi" "数据数组大小"() -> (w672:i32)
                n580 = Greater Than 0?(x=w672) -> (x > 0?=w673:bool)
                n581 = case shown="True" w673 {
                  frame False {
                  }
                  frame True {
                    n582 = while {
                      stop <- w676 stop-if-true
                      n583 = global read "全局 数据数组大小.vi" "数据数组大小"() -> (w678:i32)
                      n584 = global read "全局 小时数据发送次数.vi" "小时数据发送次数"() -> (w677:i32)
                      n585 = Decrement(x=w678) -> (x-1=w679:i32)
                      n586 = Greater Or Equal?(x=w677, y=w679) -> (x >= y?=w676:bool)
                      n587 = Get Date/Time In Seconds() -> (seconds since 1Jan1904=w686:timestamp)
                      n588 = Format Date/Time String(time format string (%c)="%Y%m%d%H%M%S%3u" ("时间格式字符串(%c)"), seconds (now)=w686) -> (date/time string=w685:string)  [unwired: 1 in]
                      n589 = Search and Replace String(input string=w685, search string="." ("搜索字符串")) -> (result string=w683:string)  [unwired: 6 in, 3 out]
                      n590 = global read "断电保存全局.vi" "MN"() -> (w682:string)
                      n591 = global read "断电保存全局.vi" "PW"() -> (w681:string)
                      n592 = call "数据编码.vi"("table输入"="3093报警信息" ("新元素/子数组"), "QN"=w683, "MN"=w682, "PW"=w681) -> ("错误常量"=w680:errorcluster, "通讯包字符串"=w674:string)  [unwired: 10 in]
                      n593 = call "通信状态入队列.vi"("错误输入（无错误）"=w680, "发送报文"=w674, "枚举"=enum16{"打开连接", "发送数据", "读取数据", "数据处理", "关闭连接"}."发送数据") -> ()  [unwired: 8 in, 1 out]
                    }
                  }
                }
              }
              frame True {
              }
            }
          }
        }
        n594 = global read "断电保存全局.vi" "仪器参数发送"() -> (w644:bool)
        n595 = case shown="True" w644 {
          tunnel: ["环境参数" ("组合框") "仪器参数" ("组合框")] -> w643
          frame False {
          }
          frame True {
          }
        }
      }
      frame "仪器参数" {
        n596 = flat-sequence {
          frame #0 {
            n597 = global write "全局 小时数据发送次数.vi" "小时数据发送次数"(0 ("小时数据发送次数")) -> ()
            n598 = global write "全局1.vi" "枚举"(enum16{"返回请求应答", "上传数据", "返回执行结果"}."上传数据" ("枚举")) -> ()
          }
          frame #1 {
            n599 = call "获取操作日志 (子VI).vi"("table输入"="仪器参数") -> ()  [unwired: 11 in]
          }
          frame #2 {
            n600 = global read "全局 数据发送重叠.vi" "掉线指示灯"() -> (w695:bool)
            n601 = Not(x=w695) -> (.not. x?=w694:bool)
            n602 = case shown="True" w694 {
              frame False {
              }
              frame True {
                n603 = global read "全局 时间2.vi" "仪器参数索引"() -> (w699:T18)
                n604 = Cluster To Array(cluster=w699) -> (array=w698:string[])
                n605 = for {
                  tunnel: [w703] -> w696 mode=indexing
                  tunnel: w698 -> [w702] mode=indexing
                  i -> [w701]
                  # "行数大于零"
                  n606 = case shown="14" w701 {
                    tunnel: [w707 w708 w709 w710 w711 w712 w713 w714 w715 w716 w717 w718 w719 w720 w721] -> w700
                    frame 0, Default {
                      n607 = global read "全局 所有参数.vi" "氨氮"() -> (w707:string[][])
                    }
                    frame 1 {
                      n608 = global read "全局 所有参数.vi" "总磷"() -> (w708:string[][])
                    }
                    frame 2 {
                      n609 = global read "全局 所有参数.vi" "总氮"() -> (w709:string[][])
                    }
                    frame 3 {
                      n610 = global read "全局 所有参数.vi" "CODMn"() -> (w710:string[][])
                    }
                    frame 4 {
                      n611 = global read "全局 所有参数.vi" "CODCr"() -> (w711:string[][])
                    }
                    frame 5 {
                      n612 = global read "全局 所有参数.vi" "DO"() -> (w712:string[][])
                    }
                    frame 6 {
                      n613 = global read "全局 所有参数.vi" "PH"() -> (w713:string[][])
                    }
                    frame 7 {
                      n614 = global read "全局 所有参数.vi" "电导率"() -> (w714:string[][])
                    }
                    frame 8 {
                      n615 = global read "全局 所有参数.vi" "水温"() -> (w715:string[][])
                    }
                    frame 9 {
                      n616 = global read "全局 所有参数.vi" "浊度"() -> (w716:string[][])
                    }
                    frame 10 {
                      n617 = global read "全局 所有参数.vi" "叶绿素"() -> (w717:string[][])
                    }
                    frame 11 {
                      n618 = global read "全局 所有参数.vi" "藻密度"() -> (w718:string[][])
                    }
                    frame 12 {
                      n619 = global read "全局 所有参数.vi" "ORP"() -> (w719:string[][])
                    }
                    frame 13 {
                      n620 = global read "全局 所有参数.vi" "氟化物"() -> (w720:string[][])
                    }
                    frame 14 {
                      n621 = global read "全局 所有参数.vi" "挥发酚"() -> (w721:string[][])
                    }
                  }
                  n622 = Array Size(array=w700) -> (size(s)=w705:i32[])
                  n623 = Index Array(array=w705) -> (element=w704:i32)  [unwired: 1 in]
                  n624 = Greater Than 0?(x=w704) -> (x > 0?=w706:bool)
                  n625 = case shown="True" w706 {
                    tunnel: w704 -> [_ _]
                    tunnel: w700 -> [_ w727]
                    tunnel: [w722 w724] -> w703
                    tunnel: w702 -> [w722 _]
                    frame False {
                    }
                    frame True {
                      # "最新时间戳加1秒"
                      n626 = Array Size(array=w727) -> (size(s)=w729:i32[])
                      n627 = Index Array(array=w729) -> (element=w728:i32)  [unwired: 1 in]
                      n628 = Decrement(x=w728) -> (x-1=w726:i32)
                      n629 = Index Array(array=w727, index (row)=w726, index (col)=0 ("禁用的索引 (列)")) -> (element=w730:string)
                      n630 = call "日期时间字符串转换分钟数加一.vi"("枚举"=enum16{"分钟数加一", "秒数加一", "小时数加一"}."秒数加一", "data[0]"=w730) -> ("日期/时间字符串"=w724:string)  [unwired: 9 in]
                    }
                  }
                }
                n631 = Array To Cluster(array=w696) -> (cluster=w697:T19)
                n632 = global write "全局 时间2.vi" "仪器参数索引"(w697) -> ()
              }
            }
          }
          frame #3 {
            n633 = global read "全局 数据发送重叠.vi" "掉线指示灯"() -> (w732:bool)
            n634 = Not(x=w732) -> (.not. x?=w731:bool)
            n635 = case shown="True" w731 {
              frame False {
              }
              frame True {
                n636 = call "3020仪器参数发送.vi"() -> ()  [unwired: 12 in]
              }
            }
          }
        }
      }
      frame "环境参数", Default {
        n637 = call "核查数据断电保存 (子VI).vi"() -> ()  [unwired: 12 in]
      }
    }
  }
  "错误输出" <- w3
